vi "aw_HeaderErrors.vi"(8 "error in":errorcluster, 10 "Response Body":string, 11 "Response Headers":string) -> (0 "error out":errorcluster, 2 "Response Body Out":string, 3 "Response Headers Out":string)   [LabVIEW 2015, in "AuraWheel.lvlib"]
uses:
  AuraWheel.lvlib
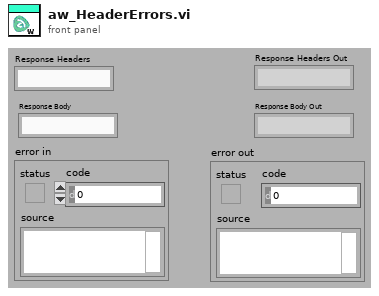
[diagram p1: front panel]
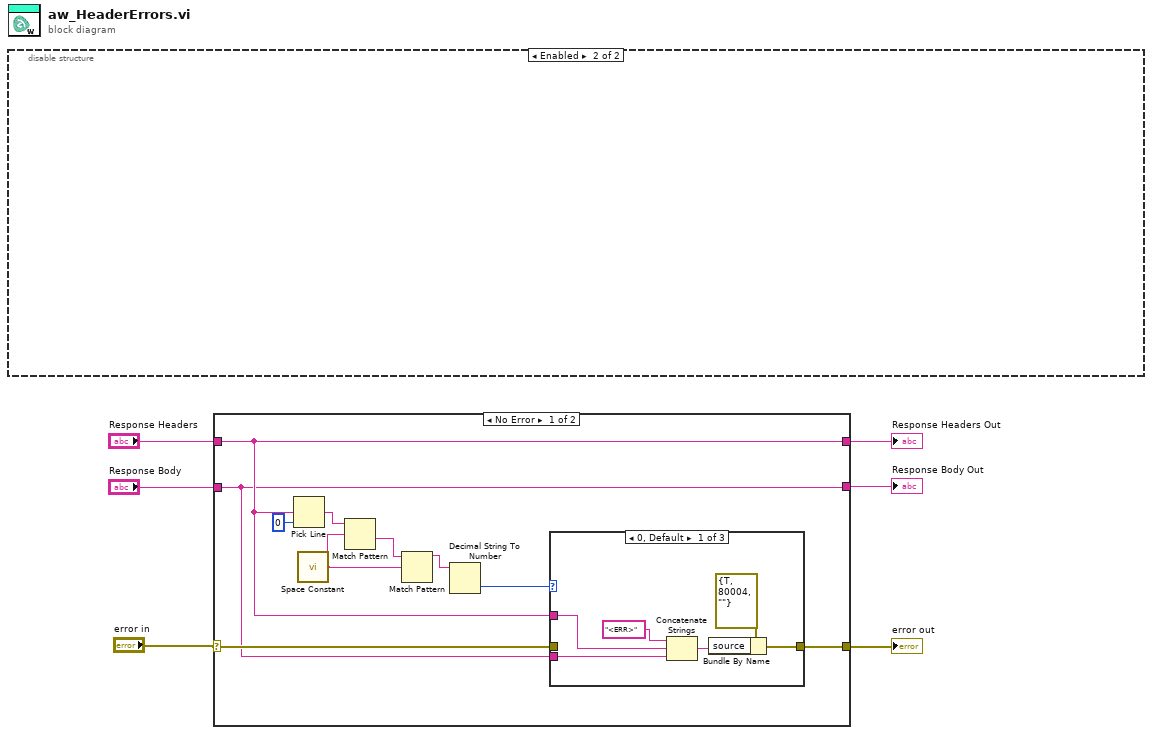
[diagram p0: block diagram]
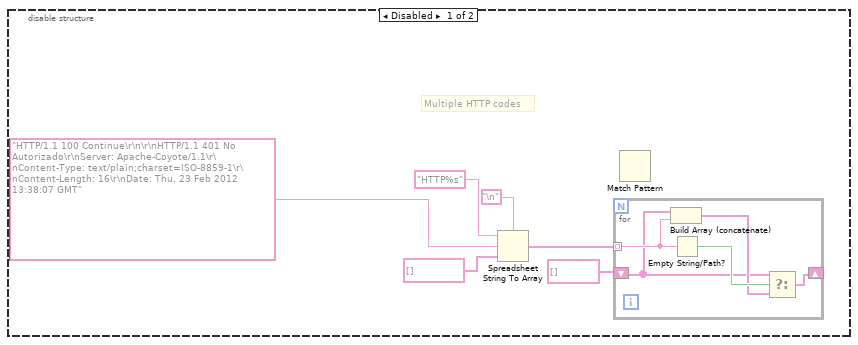
[diagram p2: hidden frame]
diagram:
  n1 = disable-structure shown="Enabled" {
    frame Disabled {
      # "Multiple HTTP codes"
      n2 = Spreadsheet String To Array(delimiter (Tab)="\n", format string="HTTP%s", spreadsheet string="HTTP/1.1 100 Continue\r\n\r\nHTTP/1.1 401 No Autorizado\r\nServer: Apache-Coyote/1.1\r\nContent-Type: text/plain;charset=ISO-8859-1\r\nContent-Length: 16\r\nDate: Thu, 23 Feb 2012 13:38:07 GMT", array type (2D Dbl)=string[] []) -> (array=w9:string[])
      n3 = for {
        tunnel: w9 -> [w16] mode=indexing
        shift-right: [w14] -> _
        shift-left: string[] [] -> [w13]
        n4 = Build Array (concatenate)(w13, w16) -> (w15:string[])
        n5 = Empty String/Path?(string/path=w16) -> (empty?=w17:bool)
        n6 = Select(t=w13, s=w17, f=w15) -> (s? t:f=w14:string[])
      }
      n7 = Match Pattern() -> ()  [unwired: 3 in, 4 out]
    }
    frame Enabled {
    }
  }
  n8 = case shown="No Error" "error in" {
    selector: "error in" -> [w21 w38]
    tunnel: [w27 w38] -> w6
    tunnel: "Response Headers" -> [w19 w37]
    tunnel: [w19 w37] -> w2
    tunnel: [w18 w36] -> w1
    tunnel: "Response Body" -> [w18 w36]
    frame No Error {
      n9 = Pick Line(multi-line string=w19, line index=0) -> (output string=w22:string)  [unwired: 1 in]
      n10 = call <vilib>:"Space Constant.vi"() -> ("String"=w24:string)
      n11 = Match Pattern(string=w22, regular expression=w24) -> (after substring=w23:string)  [unwired: 1 in, 3 out]
      n12 = Match Pattern(string=w23, regular expression=w24) -> (before substring=w26:string)  [unwired: 1 in, 3 out]
      n13 = Decimal String To Number(string=w26) -> (number=w20:i32)  [unwired: 2 in, 1 out]
      n14 = case shown="0, Default" w20 {
        tunnel: w21 -> [_ w34 w35]
        tunnel: [w30 w34 w35] -> w27
        tunnel: w19 -> [w29 _ _]
        tunnel: w18 -> [w28 _ _]
        frame 0, Default {
          n15 = Concatenate Strings("<ERR>" ("Format String"), w29, w28) -> (w32:string)
          n16 = Bundle By Name(cluster=errorcluster {"status"=TRUE, "code"=80004, "source"=""} ("error in"), "source"=w32) -> (w30:errorcluster)
        }
        frame 200..299 {
        }
        frame 100 {
        }
      }
    }
    frame Error {
    }
  }
  "error out" <- w6
  "Response Headers Out" <- w2
  "Response Body Out" <- w1
